vi "operation.vi"(9 "Return Data (T)":bool=TRUE, 10 "Command Text":string) -> (3 "Data":string[][](array[string]))   [LabVIEW 2016, in "database.lvlib"]
uses:
  database.lvlib
panel:
  out "error out":errorcluster
  in  "error in (no error)":errorcluster
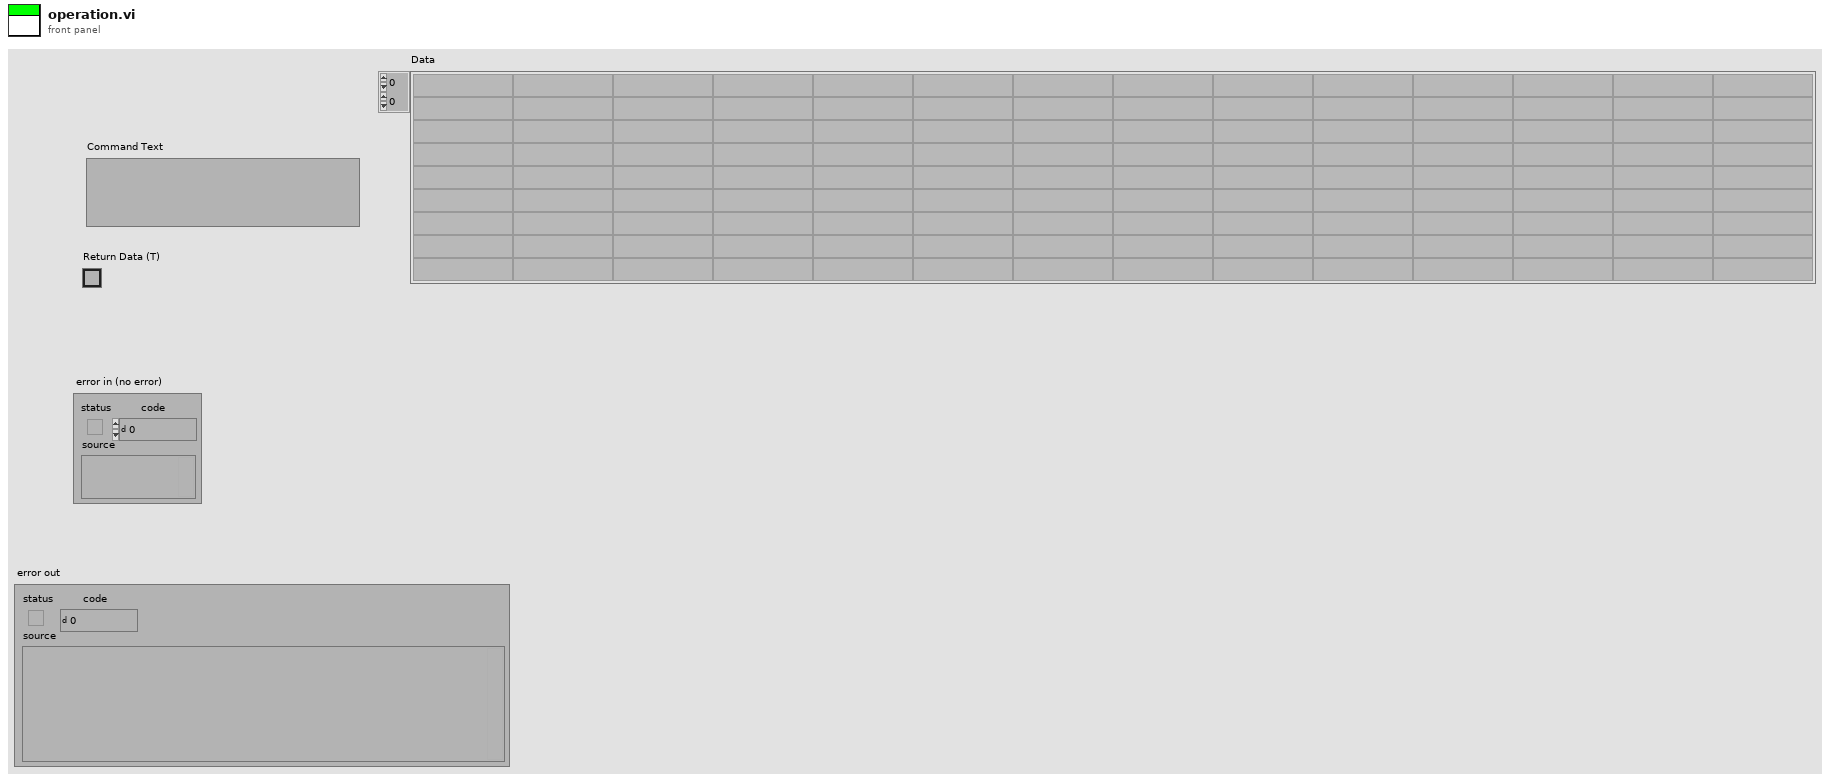
[diagram p1: front panel]
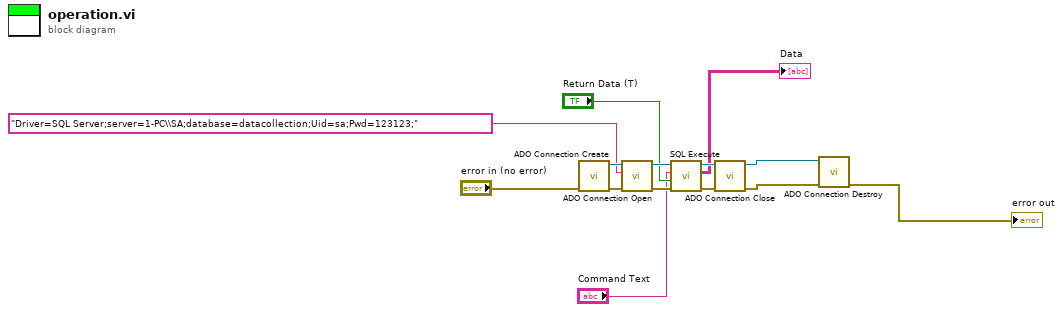
[diagram p0: block diagram]
diagram:
  n1 = call <userlib>:"ADO Connection Create.vi"("error in (no error)"="error in (no error)") -> ("error out"=w13:errorcluster, "ADODB._Connection Out"=w14:refnum<k7>)  [unwired: 9 in]
  n2 = call <userlib>:"ADO Connection Open.vi"("error in (no error)"=w13, "ConnectionString"="Driver=SQL Server;server=1-PC\\SA;database=datacollection;Uid=sa;Pwd=123123;", "ADODB._Connection In"=w14) -> ("error out"=w11:errorcluster, "ADODB._Connection Out"=w12:refnum<k7>)  [unwired: 7 in]
  n3 = call <userlib>:"SQL Execute.vi"("error in (no error)"=w11, "Return Data (T)"="Return Data (T)", "Command Text"="Command Text", "ADODB._Connection In"=w12) -> ("error out"=w9:errorcluster, "Data"=→"Data":string[][], "ADODB._Connection Out"=w10:refnum<k7>)  [unwired: 4 in, 1 out]
  n4 = call <userlib>:"ADO Connection Close.vi"("error in (no error)"=w9, "ADODB._Connection In"=w10) -> ("error out"=w7:errorcluster, "ADODB._Connection Out"=w8:refnum<k7>)  [unwired: 8 in]
  n5 = call <userlib>:"ADO Connection Destroy.vi"("error in (no error)"=w7, "ADODB._Connection In"=w8) -> ("error out"=→"error out":errorcluster)  [unwired: 9 in]
